vi "Acquisition.vi"() -> ()   [LabVIEW 2013]
panel:
  out "Go":bool
  out "Previous 2":dbl
  out "Current  2":dbl
  out "diff 2":dbl
  out "Signal 1":dynamicdata(graph)
  out "Signal 4":dynamicdata(graph)
  out "Signal 3":dynamicdata(graph)
  in  "Aquire":bool
  out "Ready":bool
  out "Signal 2":dynamicdata(graph)
  in  "stop (F)":bool
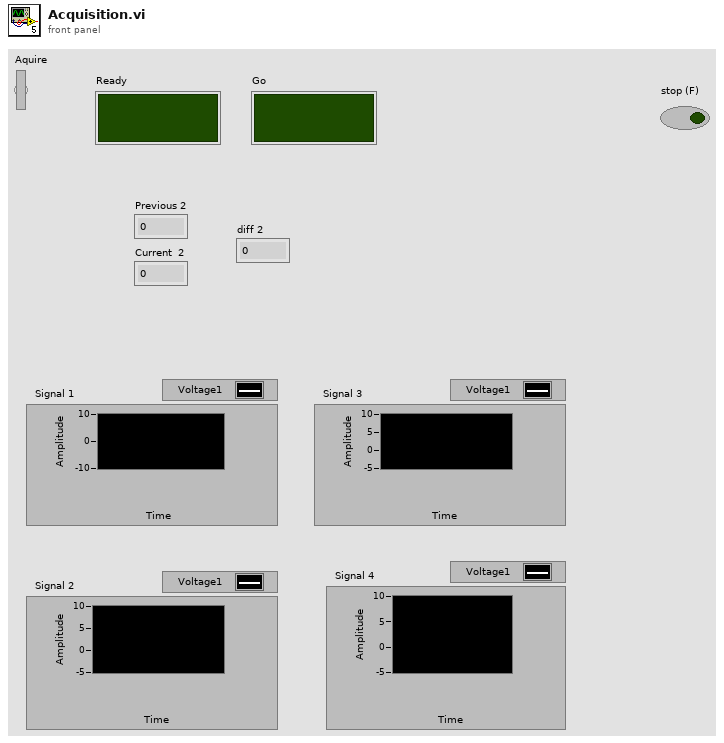
[diagram p1: front panel]
types:
  T1 = cluster{"Array":dbl[], "Array":dbl[], "Array":dbl[], "Array":dbl[]}
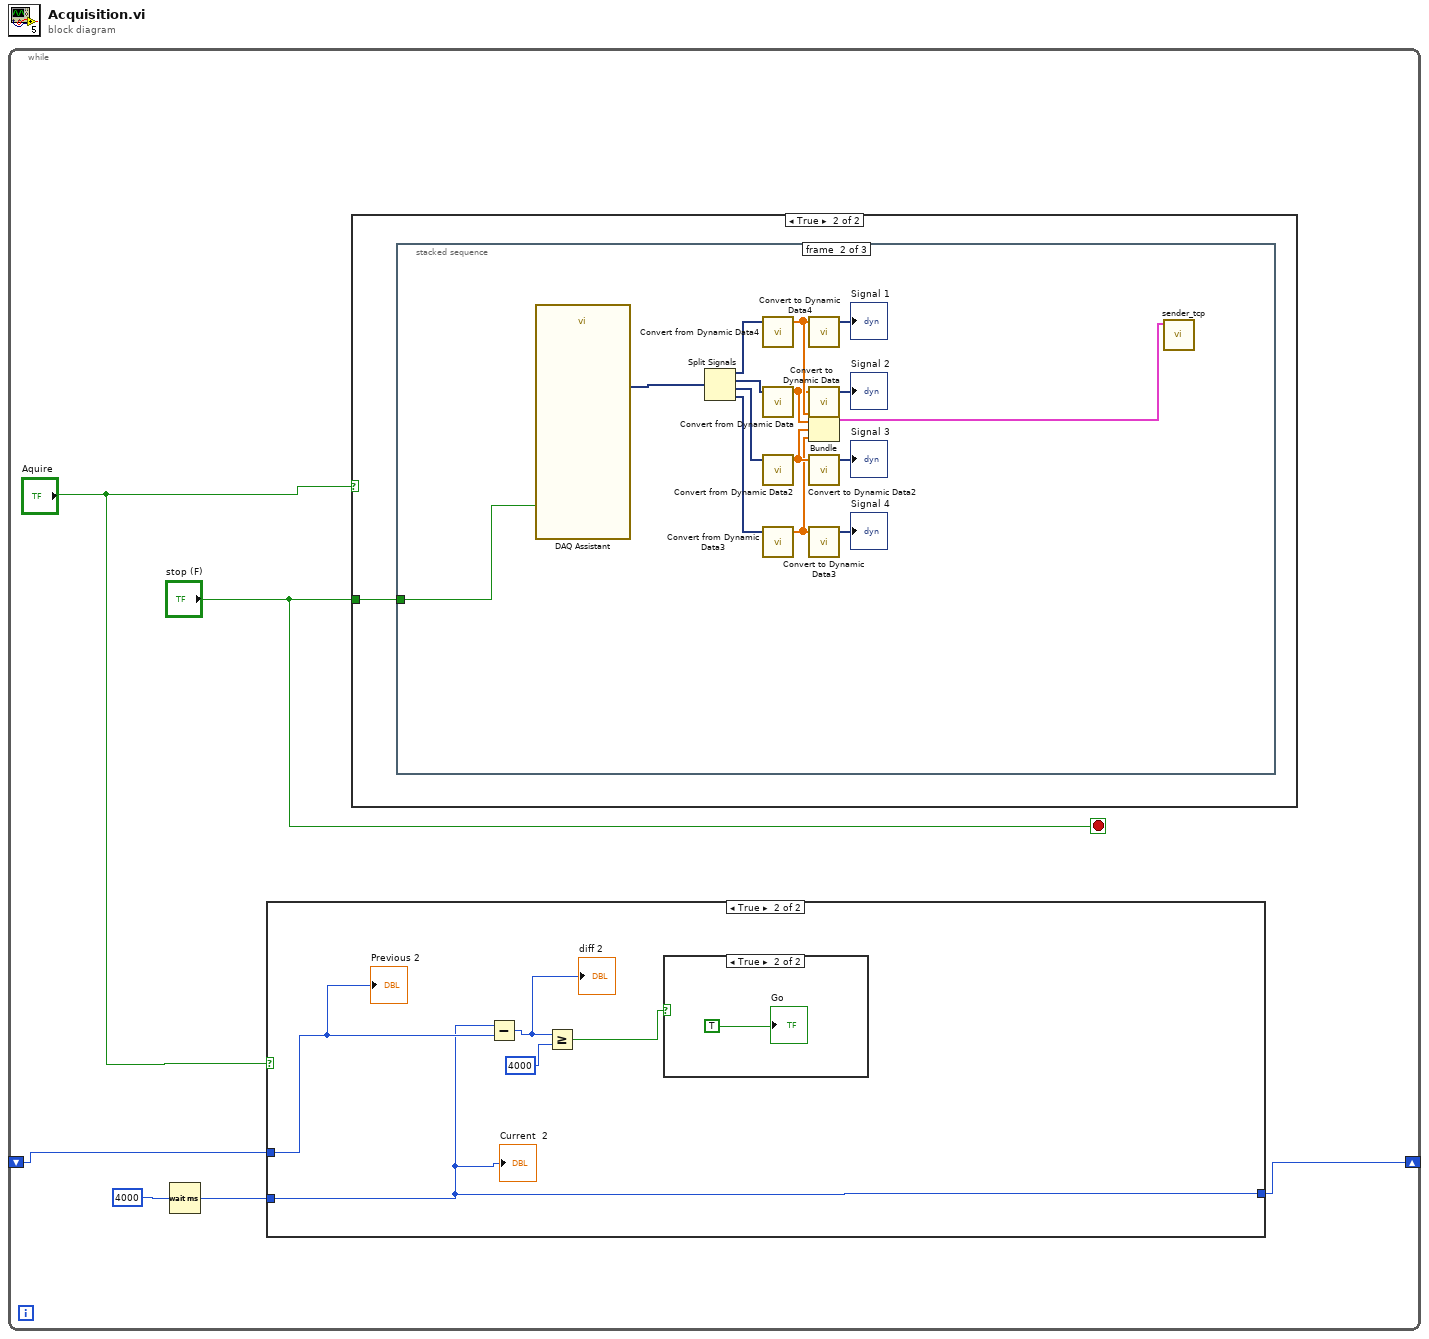
[diagram p0: block diagram]
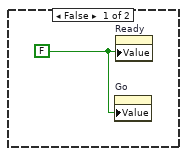
[diagram p4: hidden frame]
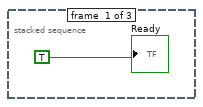
[diagram p5: hidden frame]
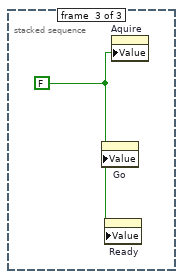
[diagram p6: hidden frame]
diagram:
  n1 = while {
    shift-right: [w3] -> _
    shift-left: _ -> [w2]
    stop <- "stop (F)" stop-if-true
    n2 = Wait (ms)(milliseconds to wait=4000) -> (millisecond timer value=w4:u32)
    n3 = case shown="True" "Aquire" {
      tunnel: [w7 w9] -> w3
      tunnel: w2 -> [_ w10]
      tunnel: w4 -> [w7 w9]
      frame False {
      }
      frame True {
        n4 = Subtract(x=w9, y=w10) -> (x-y=w8:u32)
        "diff 2" <- w8
        n5 = Greater Or Equal?(x=w8, y=u32 4000) -> (x >= y?=w11:bool)
        n6 = case shown="True" w11 {
          frame False {
          }
          frame True {
            "Go" <- TRUE
          }
        }
        "Previous 2" <- w10
        "Current  2" <- w9
      }
    }
    n7 = case shown="True" "Aquire" {
      tunnel: "stop (F)" -> [_ w15]
      frame False {
        w14 = FALSE
        n8 = property on="Go" class="Bool (strict)"("Value"=w14) -> ()  [unwired: 2 in, 2 out]
        n9 = property on="Ready" class="Bool (strict)"("Value"=w14) -> ()  [unwired: 2 in, 2 out]
      }
      frame True {
        n10 = stacked-sequence {
          tunnel: w15 -> [_ w30 _]
          frame #0 {
            "Ready" <- TRUE
          }
          frame #1 {
            n11 = call "DAQ Assistant"("stop (T)"=w30) -> ("data"=w31:dynamicdata)  [unwired: 16 in, 2 out]
            n12 = Split Signals(w31) -> (w19:dynamicdata, w20:dynamicdata, w18:dynamicdata, w17:dynamicdata)  [unwired: 4 in]
            n13 = call "Convert from Dynamic Data4"("Dynamic Data Type"=w19) -> ("Array"=w25:dbl[])  [unwired: 3 in]
            n14 = call "Convert from Dynamic Data"("Dynamic Data Type"=w20) -> ("Array"=w24:dbl[])  [unwired: 3 in]
            n15 = call "Convert from Dynamic Data2"("Dynamic Data Type"=w18) -> ("Array"=w23:dbl[])  [unwired: 3 in]
            n16 = call "Convert from Dynamic Data3"("Dynamic Data Type"=w17) -> ("Array"=w22:dbl[])  [unwired: 3 in]
            n17 = call "Convert to Dynamic Data4"("Array"=w25) -> ("Dynamic Data Type"=→"Signal 1":dynamicdata)  [unwired: 3 in]
            n18 = call "Convert to Dynamic Data"("Array"=w24) -> ("Dynamic Data Type"=→"Signal 2":dynamicdata)  [unwired: 3 in]
            n19 = Bundle("Array"=w25, "Array"=w24, "Array"=w23, "Array"=w22) -> (w21:T1)  [unwired: 1 in]
            n20 = call "Convert to Dynamic Data2"("Array"=w23) -> ("Dynamic Data Type"=→"Signal 3":dynamicdata)  [unwired: 3 in]
            n21 = call "Convert to Dynamic Data3"("Array"=w22) -> ("Dynamic Data Type"=→"Signal 4":dynamicdata)  [unwired: 3 in]
            n22 = call "sender_tcp.vi"("Cluster"=w21) -> ()  [unwired: 11 in]
          }
          frame #2 {
            w32 = FALSE
            n23 = property on="Go" class="Bool (strict)"("Value"=w32) -> ()  [unwired: 2 in, 2 out]
            n24 = property on="Ready" class="Bool (strict)"("Value"=w32) -> ()  [unwired: 2 in, 2 out]
            n25 = property on="Aquire" class="Bool (strict)"("Value"=w32) -> ()  [unwired: 2 in, 2 out]
          }
        }
      }
    }
  }
